vi "TRIGER_EDGE.vi"(0 "TRIGGER EDGE":enum32{"SLOPE RISE", "SLOPE FALL"}(radio), 1 "SOURCE":enum32{"CH 1", "CH 2", "CH 3", "CH 4"}(radio), 2 "VISA TDS1012":refnum<visa-resource-name>="GPIB0::1::INSTR") -> ()   [LabVIEW 2018]
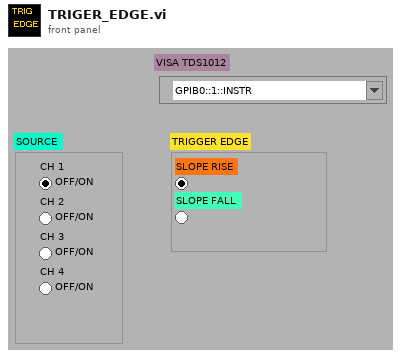
[diagram p1: front panel]
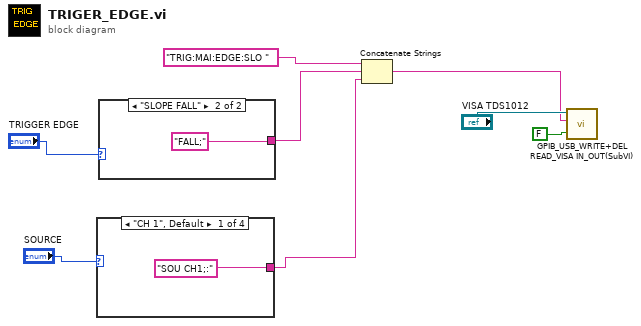
[diagram p0: block diagram]
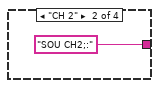
[diagram p2: hidden frame]
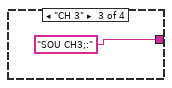
[diagram p3: hidden frame]
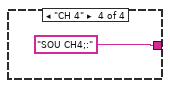
[diagram p4: hidden frame]
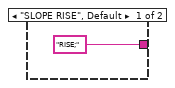
[diagram p5: hidden frame]
diagram:
  n1 = case shown="\"CH 1\", Default" "SOURCE" {
    tunnel: ["SOU CH1;:" "SOU CH2;:" "SOU CH3;:" "SOU CH4;:"] -> w1
    frame "CH 1", Default {
    }
    frame "CH 2" {
    }
    frame "CH 3" {
    }
    frame "CH 4" {
    }
  }
  n2 = case shown="\"SLOPE FALL\"" "TRIGGER EDGE" {
    tunnel: ["RISE;" "FALL;"] -> w4
    frame "SLOPE RISE", Default {
    }
    frame "SLOPE FALL" {
    }
  }
  n3 = Concatenate Strings("TRIG:MAI:EDGE:SLO ", w4, w1) -> (w3:string)
  n4 = call "GPIB_USB_WRITE+DEL READ_VISA IN_OUT(SubVI).vi"("VISA resource IN"="VISA TDS1012", "GPIB/USB WRITE"=w3, 4:FALSE ("READ GPIB")) -> ()  [unwired: 3 in, 3 out]
